vi "Record.vi"(6 "Last request":bool, 8 "error in (no error)":errorcluster, 11 "Spectrum Recorder in":refnum<class "Spectrum Recorder too.lvclass">) -> (0 "error out":errorcluster, 2 "Result":refnum<class "Acquired Result.lvclass">, 3 "Spectrum Recorder out":refnum<class "Spectrum Recorder too.lvclass">)   [LabVIEW 2016, in "Spectrum Recorder too.lvclass"]
uses:
  Spectrum Recorder too.lvclass
  C:/github/LabActor/Worker/Worker.lvclass
  C:/github/LabActor/Instrument Actor/Instrument Actor.lvclass
  NHMFL_Core/Libraries/Instruments/Results/Acquired Result/Acquired Result.lvclass
  Worker/Worker.lvclass/Worker.ctl
  Spectrum Recorder too.lvclass/Spectrum Recorder too.ctl
  Template Module/Read State.vi
  Read RP transceiver.vi
  Write RP transceiver.vi
  NHMFL_Core/Libraries/Red Pitaya/RP Core/RP Transceiver/RP Transceiver.lvclass
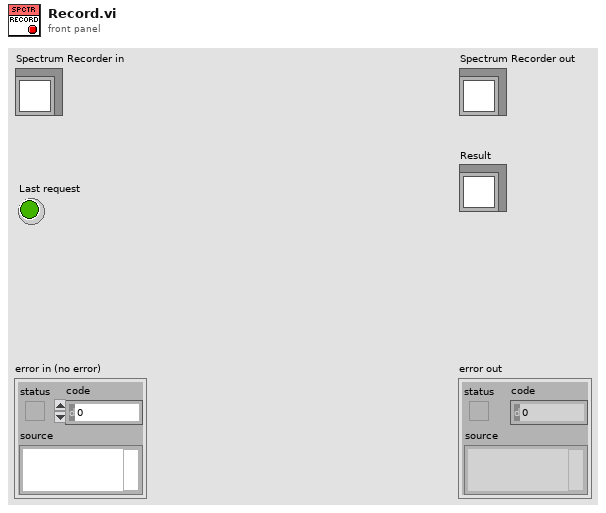
[diagram p1: front panel]
types:
  T1 = typedef "Worker State.ctl" = enum16{"Idle", "Starting", "Working", "Stopping"}
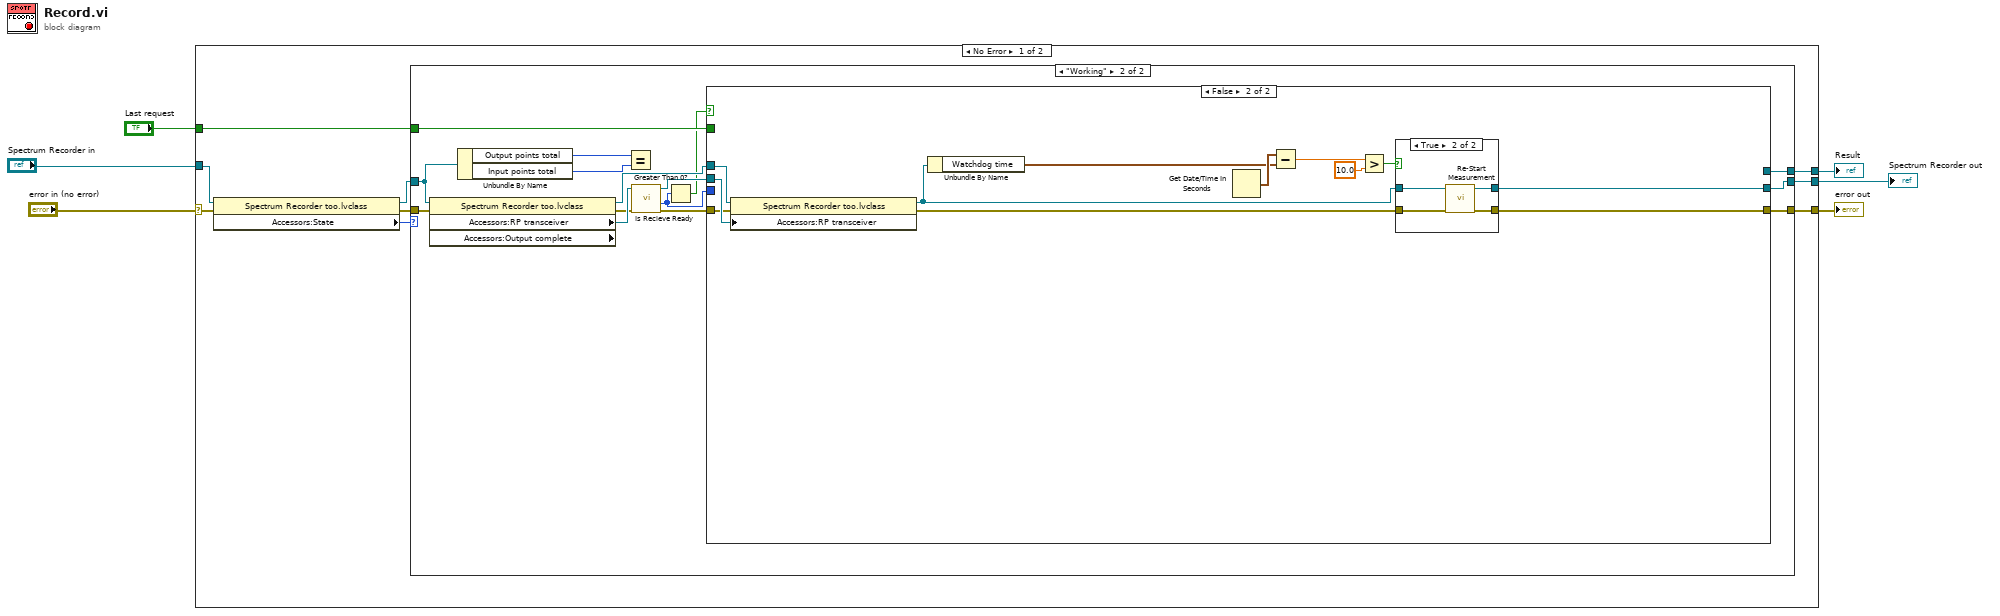
[diagram p0: block diagram]
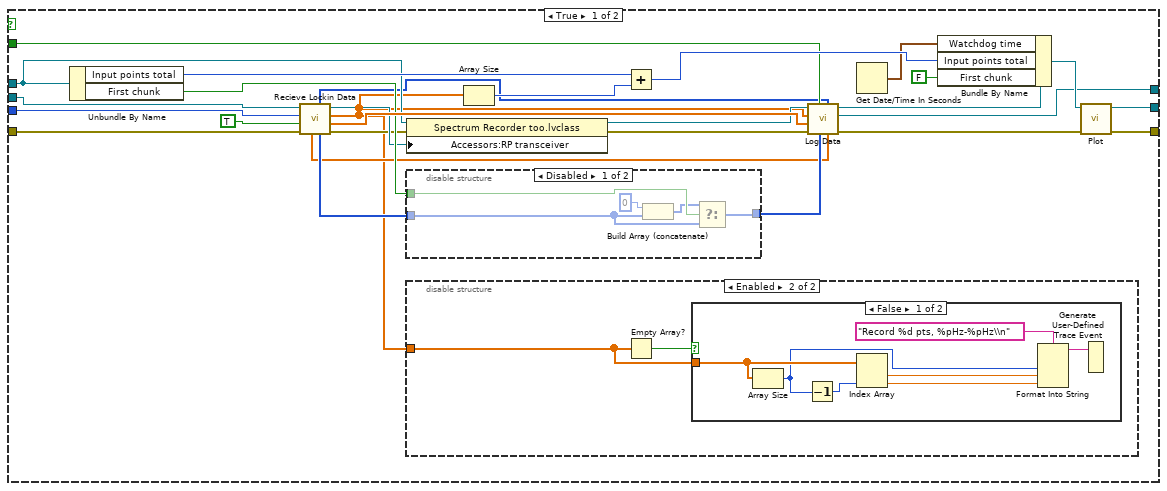
[diagram p3: hidden frame]
diagram:
  n1 = case shown="No Error" "error in (no error)" {
    selector: "error in (no error)" -> [w14 w95]
    tunnel: [w13 w95] -> w5
    tunnel: [w15 w94] -> w3
    tunnel: "Spectrum Recorder in" -> [w11 w94]
    tunnel: "Last request" -> [w8 _]
    tunnel: [w7 _] -> w1
    frame No Error {
      n2 = property class="Spectrum Recorder too.lvclass"(reference=w11, error in=w14) -> (reference out=w10:refnum<class "Spectrum Recorder too.lvclass">, error out=w12:errorcluster, "Accessors:State"=w9:T1)
      n3 = case shown="\"Working\"" w9 {
        tunnel: w10 -> [w17 w24]
        tunnel: w12 -> [w16 w27]
        tunnel: [w17 w29] -> w15
        tunnel: [w16 w30] -> w13
        tunnel: w8 -> [_ w20]
        tunnel: [_ w19] -> w7
        frame "Idle", Default {
        }
        frame "Working" {
          n4 = property class="Spectrum Recorder too.lvclass" props=["Accessors:RP transceiver", "Accessors:Output complete"](reference=w24, error in=w27) -> (reference out=w25:refnum<class "Spectrum Recorder too.lvclass">, error out=w26:errorcluster, "Accessors:RP transceiver"=w28:refnum<class "RP Transceiver.lvclass">)  [unwired: 1 out]
          n5 = Unbundle By Name(w24) -> ("Output points total"=w23:i64, "Input points total"=w22:i64)
          n6 = Equal?(x=w23, y=w22) -> ()  [unwired: 1 out]
          n7 = call-dynamic "Is Recieve Ready.vi"("error in (no error)"=w26, "RP Instrument in"=w28) -> ("error out"=w32:errorcluster, "Points in buffer"=w21:i32, "RP Instrument out"=w31:refnum<class "RP Transceiver.lvclass">)  [unwired: 6 in, 1 out]
          n8 = Greater Than 0?(x=w21) -> (x > 0?=w18:bool)
          n9 = case shown="False" w18 {
            tunnel: w32 -> [w60 w85]
            tunnel: w31 -> [w59 w86]
            tunnel: w21 -> [w58 _]
            tunnel: [w50 w77] -> w30
            tunnel: [w48 w79] -> w29
            tunnel: w25 -> [w44 w87]
            tunnel: w20 -> [w39 _]
            tunnel: [w36 _] -> w19
            frame True {
              n10 = Unbundle By Name(w44) -> ("Input points total"=w45:i64, "First chunk"=w56:bool)
              n11 = call-dynamic "Recieve Lockin Data.vi"("error in (no error)"=w60, "Force read"=TRUE, "Points to read"=w58, "RP Lockin in"=w59) -> ("error out"=w40:errorcluster, "Volatge X out"=w57:dbl[], "Frequency out"=w34:dbl[], "RP Lockin out"=w41:refnum<class "RP Transceiver.lvclass">, "Starting edges"=w51:i32[], "Ending edges"=w38:i32[], "Volatge Y out"=w37:dbl[])  [unwired: 1 in]
              n12 = property class="Spectrum Recorder too.lvclass"(reference=w44, error in=w40, "Accessors:RP transceiver"=w41) -> (reference out=w43:refnum<class "Spectrum Recorder too.lvclass">, error out=w42:errorcluster)
              n13 = disable-structure shown="Disabled" {
                disable-tunnel: w56 -> [w74 _]
                disable-tunnel: [w71 w75] -> w55
                disable-tunnel: w51 -> [w70 w75]
                frame Disabled {
                  n14 = Build Array (concatenate)(0, w70) -> (w72:i32[])
                  n15 = Select(t=w72, s=w74, f=w70) -> (s? t:f=w71:i32[])
                }
                frame Enabled {
                }
              }
              n16 = disable-structure shown="Enabled" {
                disable-tunnel: w34 -> [_ w61]
                frame Disabled {
                }
                frame Enabled {
                  n17 = Empty Array?(array=w61) -> (empty?=w62:bool)
                  n18 = case shown="False" w62 {
                    tunnel: w61 -> [w68 _]
                    frame False {
                      n19 = Array Size(array=w68) -> (size(s)=w67:i32)
                      n20 = Decrement(x=w67) -> (x-1=w66:i32)
                      n21 = Index Array(array=w68, index #2=w66) -> (element #1=w65:dbl, element #2=w64:dbl)  [unwired: 1 in]
                      n22 = Format Into String(format string="Record %d pts, %pHz-%pHz\\n", w67, w65, w64) -> (resulting string=w63:string)  [unwired: 2 in, 1 out]
                      n23 = Generate User-Defined Trace Event(2:w63) -> ()  [unwired: 1 in]
                    }
                    frame True {
                    }
                  }
                }
              }
              n24 = Array Size(array=w34) -> (size(s)=w46:i32)
              n25 = Add(x=w45, y=w46) -> (x+y=w47:i64)
              n26 = call-dynamic "Log Data.vi"("Volatge Y"=w37, "Ending edges"=w38, "Starting edges"=w55, "Last request"=w39, "error in (no error)"=w42, "Volatge X"=w57, "Frequency"=w34, "Spectrum Recorder in"=w43) -> ("error out"=w53:errorcluster, "Result"=w36:refnum<class "Acquired Result.lvclass">, "Spectrum Recorder out"=w54:refnum<class "Spectrum Recorder too.lvclass">)  [unwired: 1 in]
              n27 = Get Date/Time In Seconds() -> (seconds since 1Jan1904=w33:timestamp)
              n28 = Bundle By Name(cluster=w54, "Watchdog time"=w33, "Input points total"=w47, "First chunk"=FALSE) -> (w49:refnum<class "Spectrum Recorder too.lvclass">)
              n29 = call-dynamic "Plot.vi"("error in (no error)"=w53, "Spectrum Recorder in"=w49) -> ("error out"=w50:errorcluster, "Spectrum Recorder out"=w48:refnum<class "Spectrum Recorder too.lvclass">)  [unwired: 8 in]
            }
            frame False {
              n30 = property class="Spectrum Recorder too.lvclass"(reference=w87, error in=w85, "Accessors:RP transceiver"=w86) -> (reference out=w80:refnum<class "Spectrum Recorder too.lvclass">, error out=w78:errorcluster)
              n31 = Unbundle By Name(w80) -> ("Watchdog time"=w83:timestamp)
              n32 = Get Date/Time In Seconds() -> (seconds since 1Jan1904=w84:timestamp)
              n33 = Subtract(x=w84, y=w83) -> (x-y=w82:dbl)
              n34 = Greater?(x=w82, y=10.0) -> (0:w76:bool)
              n35 = case shown="True" w76 {
                tunnel: w80 -> [w89 w93]
                tunnel: [w89 w92] -> w79
                tunnel: w78 -> [w88 w91]
                tunnel: [w88 w90] -> w77
                frame False {
                }
                frame True {
                  n36 = call-dynamic "Re-Start Measurement.vi"("error in (no error)"=w91, "Spectrum Recorder too in"=w93) -> ("error out"=w90:errorcluster, "Spectrum Recorder too out"=w92:refnum<class "Spectrum Recorder too.lvclass">)  [unwired: 8 in]
                }
              }
            }
          }
        }
      }
    }
    frame Error {
    }
  }
  "error out" <- w5
  "Spectrum Recorder out" <- w3
  "Result" <- w1
